vi "niDDC Fetch.vi"(8 "error in (no error)":errorcluster, 9 "seconds to read (-1:all)":dbl=0.001 format="%#_13p", 11 "Class in":refnum<class "7976R_v1.lvclass">) -> (0 "error out":errorcluster, 1 "Timeout?":bool=TRUE, 2 "Complex wfm out":waveform(cdb), 3 "Class out":refnum<class "7976R_v1.lvclass">)   [LabVIEW 2015, in "7976R_v1.lvclass"]
uses:
  <userlib>/SE-APP-Receiver/NI5772/7976R_v1/7976R_v1.lvclass
  <userlib>/SE-APP-Receiver/NI5772/7976R_v1/7976R_v1.lvclass/7976R_v1.ctl
  <vilib>/Utility/error.llb/Error Cluster From Error Code.vi
  <vilib>/rvi/errors/niLvFpgaAdjustHostInterfaceError.vi
  <vilib>/rvi/interface/nirviMethod/nirviMethod.xnode
  <userlib>/SE-APP-Receiver/NI5772/7976R_v1/Private/FPGA VI Reference_DDC_v1.8.ctl
  <vilib>/FPGAPlugInAG/Dynamic/niLvFpga_ReadFifo_Dynamic.vi
  <vilib>/rvi/errors/niLvFpgaMergeErrorWithErrorCode.vi
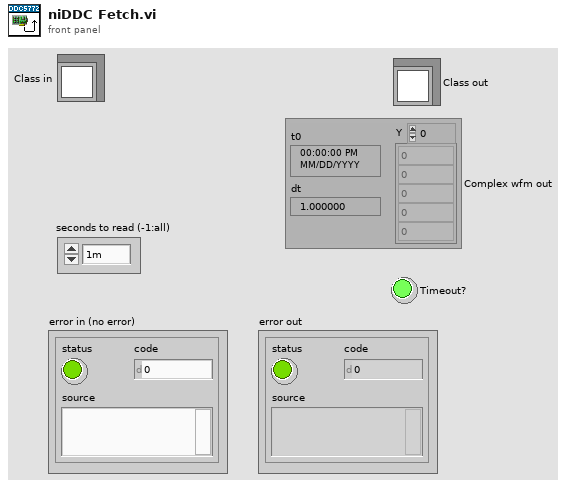
[diagram p1: front panel]
types:
  T1 = typedef "7976R_v1.lvclass/FPGA VI Reference_DDC_v1.8.ctl" = refnum<k20>
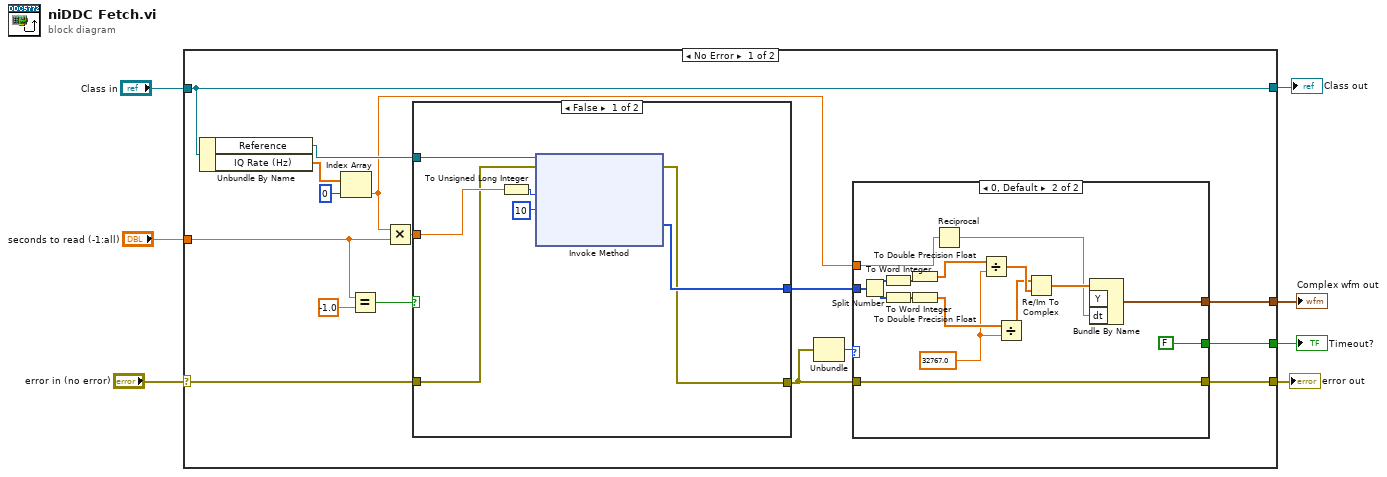
[diagram p0: block diagram]
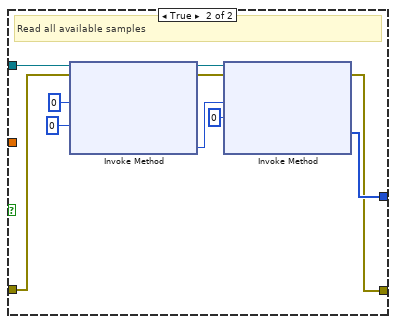
[diagram p2: hidden frame]
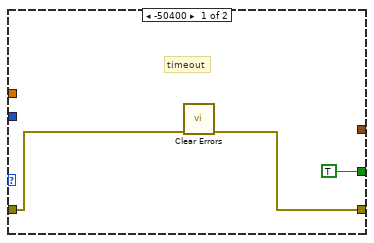
[diagram p3: hidden frame]
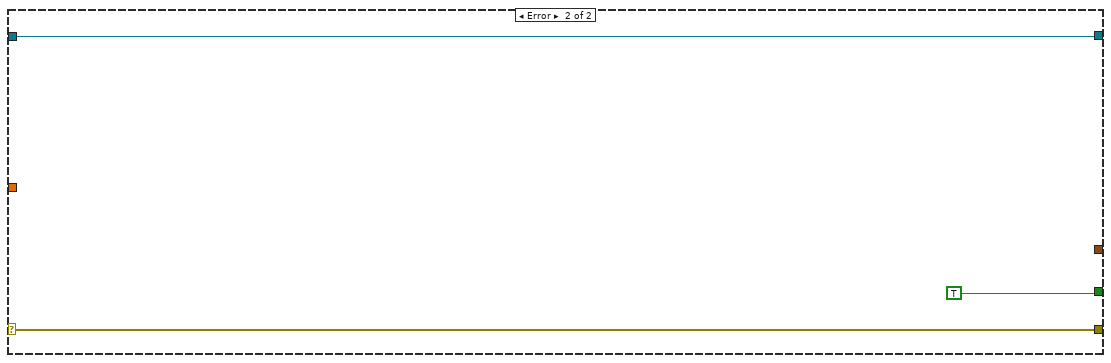
[diagram p4: hidden frame]
diagram:
  n1 = case shown="No Error" "error in (no error)" {
    selector: "error in (no error)" -> [w13 w62]
    tunnel: [w14 w62] -> w7
    tunnel: "Class in" -> [w20 w61]
    tunnel: [w20 w61] -> w4
    tunnel: "seconds to read (-1:all)" -> [w10 _]
    tunnel: [w12 _] -> w2
    tunnel: [w11 TRUE] -> w1
    frame No Error {
      n2 = Unbundle By Name(w20) -> ("Reference"=w19:T1, "IQ Rate (Hz)"=w18:dbl[])
      n3 = Index Array(array=w18, index=0) -> (element=w15:dbl)
      n4 = Equal?(x=w10, y=-1.0) -> (x = y?=w8:bool)
      n5 = Multiply(x=w15, y=w10) -> (x*y=w16:dbl)
      n6 = case shown="False" w8 {
        tunnel: [w30 w33] -> w22
        tunnel: [w29 w32] -> w21
        tunnel: w19 -> [w26 w38]
        tunnel: w16 -> [w25 _]
        tunnel: w13 -> [w24 w31]
        frame False {
          n7 = To Unsigned Long Integer(number=w25) -> (unsigned 32bit integer=w28:u32)
          n8 = xnode "Invoke Method"("FPGA VI Reference In"=w26, "error in"=w24, "Number of Elements"=w28, "Timeout (ms)"=10) -> ("error out"=w29:errorcluster, "Data"=w30:u32[])  [unwired: 2 out]
        }
        frame True {
          # "Read all available samples"
          n9 = xnode "Invoke Method"("FPGA VI Reference In"=w38, "error in"=w31, "Number of Elements"=u32 0, "Timeout (ms)"=0) -> ("FPGA VI Reference Out"=w40:T1, "error out"=w39:errorcluster, "Elements Remaining"=w35:u32)  [unwired: 1 out]
          n10 = xnode "Invoke Method"("FPGA VI Reference In"=w40, "error in"=w39, "Number of Elements"=w35, "Timeout (ms)"=0) -> ("error out"=w32:errorcluster, "Data"=w33:u32[])  [unwired: 2 out]
        }
      }
      n11 = Unbundle(w21) -> ("code"=w23:i32)  [unwired: 2 out]
      n12 = case shown="0, Default" w23 {
        tunnel: w22 -> [_ w54]
        tunnel: w21 -> [w43 w46]
        tunnel: [w42 w46] -> w14
        tunnel: w15 -> [_ w47]
        tunnel: [_ w45] -> w12
        tunnel: [TRUE FALSE] -> w11
        frame -50400 {
          # "timeout"
          n13 = call <vilib>:"Clear Errors.vi"("error in (no error)"=w43) -> ("error out"=w42:errorcluster)  [unwired: 5 in, 1 out]
        }
        frame 0, Default {
          w51 = 32767.0
          n14 = Split Number(x=w54) -> (hi(x)=w59:u16[], lo(x)=w58:u16[])
          n15 = To Word Integer(number=w59) -> (16bit integer=w57:i16[])
          n16 = To Word Integer(number=w58) -> (16bit integer=w56:i16[])
          n17 = To Double Precision Float(number=w57) -> (double precision float=w53:dbl[])
          n18 = To Double Precision Float(number=w56) -> (double precision float=w52:dbl[])
          n19 = Reciprocal(x=w47) -> (1/x=w48:dbl)
          n20 = Divide(x=w53, y=w51) -> (x/y=w50:dbl[])
          n21 = Divide(x=w52, y=w51) -> (x/y=w49:dbl[])
          n22 = Re/Im To Complex(1:w50, 2:w49) -> (0:w55:cdb[])
          n23 = Bundle By Name("Y"=w55, "dt"=w48) -> (w45:waveform(cdb))  [unwired: 1 in]
        }
      }
    }
    frame Error {
    }
  }
  "error out" <- w7
  "Class out" <- w4
  "Complex wfm out" <- w2
  "Timeout?" <- w1
